vi "Register gRPC Messages.vi"(8 "error in (no error)":errorcluster, 11 "gRPC ID":T1) -> (0 "error out":errorcluster, 3 "gRPC ID Out":T1)   [LabVIEW 2021, in "CIF_PluginLoader_server.lvlib"]
uses:
  CIF_PluginLoader_server.lvlib
  <vilib>/gRPC/LabVIEW gRPC Library/Shared/grpcId.ctl
  <vilib>/gRPC/LabVIEW gRPC Library/Server API/typeDefs/Enum Metadata.ctl
  <vilib>/gRPC/LabVIEW gRPC Library/Server API/typeDefs/Message Metadata.ctl
  <vilib>/gRPC/LabVIEW gRPC Library/Server API/typeDefs/Message Element Metadata.ctl
  <vilib>/gRPC/LabVIEW gRPC Library/Server API/typeDefs/Message Element Type.ctl
  <vilib>/gRPC/LabVIEW gRPC Library/grpc-lvsupport-release.lvlib
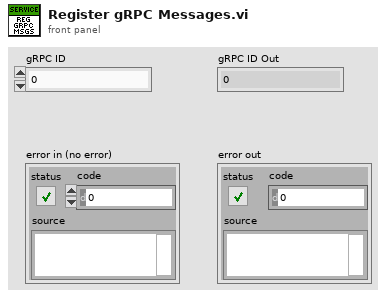
[diagram p1: front panel]
types:
  T1 = typedef "grpc-lvsupport-release.lvlib/grpcId.ctl" = u64
  T2 = typedef "grpc-lvsupport-release.lvlib/Enum Metadata.ctl" = cluster{"Version":i32, "Name":string, "Type Url":string, "Enum Values":string, "Allow Alias":bool}
  T3 = typedef "grpc-lvsupport-release.lvlib/Message Metadata.ctl" = cluster{"Version":i32, "Name":string, "Type Url":string, "Elements":T4[], "Has Oneof":bool}
  T4 = typedef "grpc-lvsupport-release.lvlib/Message Element Metadata.ctl" = cluster{"Field Name":string, "Embedded Message Name":string, "Protobuf Index":i32, "MessageElementType":T5, "Repeated":bool, "Is in Oneof":bool, "Oneof Container Name":string}
  T5 = typedef "grpc-lvsupport-release.lvlib/Message Element Type.ctl" = enum32{"Int32Value", "FloatValue", "DoubleValue", "BoolValue", "StringValue", "MessageValue", "Int64Value", "UInt32Value", "UInt64Value", "EnumValue", "Bytes", "Fixed64", "Fixed32", "SFixed64", "SFixed32", "SInt64", "SInt32"}
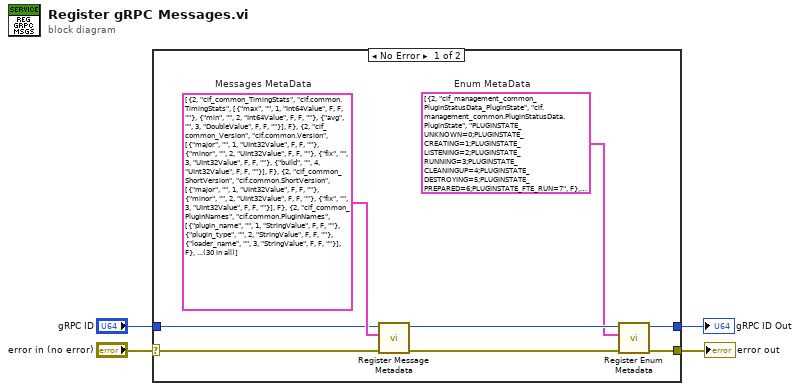
[diagram p0: block diagram]
diagram:
  n1 = case shown="No Error" "error in (no error)" {
    selector: "error in (no error)" -> [w10 w13]
    tunnel: [w9 w12] -> w2
    tunnel: [w6 w13] -> w1
    tunnel: "gRPC ID" -> [w9 w12]
    frame No Error {
      w5 = T2[] [{"Version"=2, "Name"="cif_management_common_PluginStatusData_PluginState", "Type Url"="cif.management_common.PluginStatusData.PluginState", "Enum Values"="PLUGINSTATE_UNKNOWN=0;PLUGINSTATE_CREATING=1;PLUGINSTATE_LISTENING=2;PLUGINSTATE_RUNNING=3;PLUGINSTATE_CLEANINGUP=4;PLUGINSTATE_DESTROYING=5;PLUGINSTATE_PREPARED=6;PLUGINSTATE_FTE_RUN=7", "Allow Alias"=FALSE}, {"Version"=2, "Name"="cif_management_common_ChannelDirection", "Type Url"="cif.management_common.ChannelDirection", "Enum Values"="CHANNELDIRECTION_UNKNOWN=0;CHANNELDIRECTION_PUBLISHER=1;CHANNELDIRECTION_SUBSCRIBER=2", "Allow Alias"=FALSE}, {"Version"=2, "Name"="cif_management_common_ChannelPattern", "Type Url"="cif.management_common.ChannelPattern", "Enum Values"="CHANNELPATTERN_UNKNOWN=0;CHANNELPATTERN_TAG=1;CHANNELPATTERN_FIFO=2;CHANNELPATTERN_MULTIFIFO=3;CHANNELPATTERN_BACKPRESSUREFIFO=4", "Allow Alias"=FALSE}, {"Version"=2, "Name"="cif_management_common_LoaderType", "Type Url"="cif.management_common.LoaderType", "Enum Values"="LOADERTYPE_UNKNOWN=0;LOADERTYPE_LABVIEW=1", "Allow Alias"=FALSE}]  # Enum MetaData
      w11 = T3[] [{"Version"=2, "Name"="cif_common_TimingStats", "Type Url"="cif.common.TimingStats", "Elements"=[{"Field Name"="max", "Embedded Message Name"="", "Protobuf Index"=1, "MessageElementType"=enum."Int64Value", "Repeated"=FALSE, "Is in Oneof"=FALSE, "Oneof Container Name"=""}, {"Field Name"="min", "Embedded Message Name"="", "Protobuf Index"=2, "MessageElementType"=enum."Int64Value", "Repeated"=FALSE, "Is in Oneof"=FALSE, "Oneof Container Name"=""}, {"Field Name"="avg", "Embedded Message Name"="", "Protobuf Index"=3, "MessageElementType"=enum."DoubleValue", "Repeated"=FALSE, "Is in Oneof"=FALSE, "Oneof Container Name"=""}], "Has Oneof"=FALSE}, {"Version"=2, "Name"="cif_common_Version", "Type Url"="cif.common.Version", "Elements"=[{"Field Name"="major", "Embedded Message Name"="", "Protobuf Index"=1, "MessageElementType"=enum."UInt32Value", "Repeated"=FALSE, "Is in Oneof"=FALSE, "Oneof Container Name"=""}, {"Field Name"="minor", "Embedded Message Name"="", "Protobuf Index"=2, "MessageElementType"=enum."UInt32Value", "Repeated"=FALSE, "Is in Oneof"=FALSE, "Oneof Container Name"=""}, {"Field Name"="fix", "Embedded Message Name"="", "Protobuf Index"=3, "MessageElementType"=enum."UInt32Value", "Repeated"=FALSE, "Is in Oneof"=FALSE, "Oneof Container Name"=""}, {"Field Name"="build", "Embedded Message Name"="", "Protobuf Index"=4, "MessageElementType"=enum."UInt32Value", "Repeated"=FALSE, "Is in Oneof"=FALSE, "Oneof Container Name"=""}], "Has Oneof"=FALSE}, {"Version"=2, "Name"="cif_common_ShortVersion", "Type Url"="cif.common.ShortVersion", "Elements"=[{"Field Name"="major", "Embedded Message Name"="", "Protobuf Index"=1, "MessageElementType"=enum."UInt32Value", "Repeated"=FALSE, "Is in Oneof"=FALSE, "Oneof Container Name"=""}, {"Field Name"="minor", "Embedded Message Name"="", "Protobuf Index"=2, "MessageElementType"=enum."UInt32Value", "Repeated"=FALSE, "Is in Oneof"=FALSE, "Oneof Container Name"=""}, {"Field Name"="fix", "Embedded Message Name"="", "Protobuf Index"=3, "MessageElementType"=enum."UInt32Value", "Repeated"=FALSE, "Is in Oneof"=FALSE, "Oneof Container Name"=""}], "Has Oneof"=FALSE}, {"Version"=2, "Name"="cif_common_PluginNames", "Type Url"="cif.common.PluginNames", "Elements"=[{"Field Name"="plugin_name", "Embedded Message Name"="", "Protobuf Index"=1, "MessageElementType"=enum."StringValue", "Repeated"=FALSE, "Is in Oneof"=FALSE, "Oneof Container Name"=""}, {"Field Name"="plugin_type", "Embedded Message Name"="", "Protobuf Index"=2, "MessageElementType"=enum."StringValue", "Repeated"=FALSE, "Is in Oneof"=FALSE, "Oneof Container Name"=""}, {"Field Name"="loader_name", "Embedded Message Name"="", "Protobuf Index"=3, "MessageElementType"=enum."StringValue", "Repeated"=FALSE, "Is in Oneof"=FALSE, "Oneof Container Name"=""}], "Has Oneof"=FALSE}, {"Version"=2, "Name"="cif_common_Status", "Type Url"="cif.common.Status", "Elements"=[{"Field Name"="code", "Embedded Message Name"="", "Protobuf Index"=1, "MessageElementType"=enum."Int32Value", "Repeated"=FALSE, "Is in Oneof"=FALSE, "Oneof Container Name"=""}, {"Field Name"="message", "Embedded Message Name"="", "Protobuf Index"=2, "MessageElementType"=enum."StringValue", "Repeated"=FALSE, "Is in Oneof"=FALSE, "Oneof Container Name"=""}], "Has Oneof"=FALSE}, {"Version"=2, "Name"="cif_common_Empty", "Type Url"="cif.common.Empty", "Elements"=[], "Has Oneof"=FALSE}, {"Version"=2, "Name"="cif_pluginloader_LoadPluginRequest", "Type Url"="cif.pluginloader.LoadPluginRequest", "Elements"=[{"Field Name"="plugin_name", "Embedded Message Name"="", "Protobuf Index"=1, "MessageElementType"=enum."StringValue", "Repeated"=FALSE, "Is in Oneof"=FALSE, "Oneof Container Name"=""}, {"Field Name"="path", "Embedded Message Name"="", "Protobuf Index"=2, "MessageElementType"=enum."StringValue", "Repeated"=FALSE, "Is in Oneof"=FALSE, "Oneof Container Name"=""}], "Has Oneof"=FALSE}, {"Version"=2, "Name"="cif_pluginloader_LoadPluginResponse", "Type Url"="cif.pluginloader.LoadPluginResponse", "Elements"=[{"Field Name"="status", "Embedded Message Name"="cif_common_Status", "Protobuf Index"=1, "MessageElementType"=enum."MessageValue", "Repeated"=FALSE, "Is in Oneof"=FALSE, "Oneof Container Name"=""}], "Has Oneof"=FALSE}, {"Version"=2, "Name"="cif_pluginloader_AbortPluginRequest", "Type Url"="cif.pluginloader.AbortPluginRequest", "Elements"=[{"Field Name"="plugin_name", "Embedded Message Name"="", "Protobuf Index"=1, "MessageElementType"=enum."StringValue", "Repeated"=FALSE, "Is in Oneof"=FALSE, "Oneof Container Name"=""}], "Has Oneof"=FALSE}, {"Version"=2, "Name"="cif_pluginloader_AbortPluginResponse", "Type Url"="cif.pluginloader.AbortPluginResponse", "Elements"=[{"Field Name"="status", "Embedded Message Name"="cif_common_Status", "Protobuf Index"=1, "MessageElementType"=enum."MessageValue", "Repeated"=FALSE, "Is in Oneof"=FALSE, "Oneof Container Name"=""}], "Has Oneof"=FALSE}, {"Version"=2, "Name"="cif_pluginloader_DestroyRequest", "Type Url"="cif.pluginloader.DestroyRequest", "Elements"=[], "Has Oneof"=FALSE}, {"Version"=2, "Name"="cif_pluginloader_DestroyResponse", "Type Url"="cif.pluginloader.DestroyResponse", "Elements"=[], "Has Oneof"=FALSE}, {"Version"=2, "Name"="cif_pluginloader_PingRequest", "Type Url"="cif.pluginloader.PingRequest", "Elements"=[], "Has Oneof"=FALSE}, {"Version"=2, "Name"="cif_pluginloader_PingResponse", "Type Url"="cif.pluginloader.PingResponse", "Elements"=[{"Field Name"="loader_info", "Embedded Message Name"="cif_management_common_LoaderInfoFull", "Protobuf Index"=1, "MessageElementType"=enum."MessageValue", "Repeated"=FALSE, "Is in Oneof"=FALSE, "Oneof Container Name"=""}], "Has Oneof"=FALSE}, {"Version"=2, "Name"="cif_pluginloader_DiscoverRequest", "Type Url"="cif.pluginloader.DiscoverRequest", "Elements"=[{"Field Name"="update_metadata", "Embedded Message Name"="", "Protobuf Index"=1, "MessageElementType"=enum."BoolValue", "Repeated"=FALSE, "Is in Oneof"=FALSE, "Oneof Container Name"=""}], "Has Oneof"=FALSE}, {"Version"=2, "Name"="cif_pluginloader_DiscoveredPlugin", "Type Url"="cif.pluginloader.DiscoveredPlugin", "Elements"=[{"Field Name"="file_path", "Embedded Message Name"="", "Protobuf Index"=1, "MessageElementType"=enum."StringValue", "Repeated"=FALSE, "Is in Oneof"=FALSE, "Oneof Container Name"=""}, {"Field Name"="file_name", "Embedded Message Name"="", "Protobuf Index"=2, "MessageElementType"=enum."StringValue", "Repeated"=FALSE, "Is in Oneof"=FALSE, "Oneof Container Name"=""}, {"Field Name"="plugin_type", "Embedded Message Name"="", "Protobuf Index"=3, "MessageElementType"=enum."StringValue", "Repeated"=FALSE, "Is in Oneof"=FALSE, "Oneof Container Name"=""}, {"Field Name"="plugin_version", "Embedded Message Name"="cif_common_Version", "Protobuf Index"=4, "MessageElementType"=enum."MessageValue", "Repeated"=FALSE, "Is in Oneof"=FALSE, "Oneof Container Name"=""}, {"Field Name"="plugin_metadata", "Embedded Message Name"="cif_management_common_PluginMetadata", "Protobuf Index"=5, "MessageElementType"=enum."MessageValue", "Repeated"=FALSE, "Is in Oneof"=FALSE, "Oneof Container Name"=""}, {"Field Name"="relative_path", "Embedded Message Name"="", "Protobuf Index"=6, "MessageElementType"=enum."StringValue", "Repeated"=TRUE, "Is in Oneof"=FALSE, "Oneof Container Name"=""}], "Has Oneof"=FALSE}, {"Version"=2, "Name"="cif_pluginloader_DiscoverResponse", "Type Url"="cif.pluginloader.DiscoverResponse", "Elements"=[{"Field Name"="discovered_plugins", "Embedded Message Name"="cif_pluginloader_DiscoveredPlugin", "Protobuf Index"=1, "MessageElementType"=enum."MessageValue", "Repeated"=TRUE, "Is in Oneof"=FALSE, "Oneof Container Name"=""}, {"Field Name"="status", "Embedded Message Name"="cif_common_Status", "Protobuf Index"=2, "MessageElementType"=enum."MessageValue", "Repeated"=FALSE, "Is in Oneof"=FALSE, "Oneof Container Name"=""}], "Has Oneof"=FALSE}, {"Version"=2, "Name"="cif_management_common_PluginMetadata", "Type Url"="cif.management_common.PluginMetadata", "Elements"=[{"Field Name"="description", "Embedded Message Name"="", "Protobuf Index"=1, "MessageElementType"=enum."StringValue", "Repeated"=FALSE, "Is in Oneof"=FALSE, "Oneof Container Name"=""}, {"Field Name"="history", "Embedded Message Name"="", "Protobuf Index"=2, "MessageElementType"=enum."StringValue", "Repeated"=FALSE, "Is in Oneof"=FALSE, "Oneof Container Name"=""}, {"Field Name"="author", "Embedded Message Name"="", "Protobuf Index"=3, "MessageElementType"=enum."StringValue", "Repeated"=FALSE, "Is in Oneof"=FALSE, "Oneof Container Name"=""}], "Has Oneof"=FALSE}, {"Version"=2, "Name"="cif_management_common_Channels", "Type Url"="cif.management_common.Channels", "Elements"=[{"Field Name"="channels", "Embedded Message Name"="cif_management_common_Channel", "Protobuf Index"=1, "MessageElementType"=enum."MessageValue", "Repeated"=TRUE, "Is in Oneof"=FALSE, "Oneof Container Name"=""}], "Has Oneof"=FALSE}, {"Version"=2, "Name"="cif_management_common_Channel", "Type Url"="cif.management_common.Channel", "Elements"=[{"Field Name"="name", "Embedded Message Name"="", "Protobuf Index"=1, "MessageElementType"=enum."StringValue", "Repeated"=FALSE, "Is in Oneof"=FALSE, "Oneof Container Name"=""}, {"Field Name"="direction", "Embedded Message Name"="cif_management_common_ChannelDirection", "Protobuf Index"=2, "MessageElementType"=enum."EnumValue", "Repeated"=FALSE, "Is in Oneof"=FALSE, "Oneof Container Name"=""}, {"Field Name"="type", "Embedded Message Name"="", "Protobuf Index"=3, "MessageElementType"=enum."StringValue", "Repeated"=FALSE, "Is in Oneof"=FALSE, "Oneof Container Name"=""}, {"Field Name"="custom_config", "Embedded Message Name"="", "Protobuf Index"=4, "MessageElementType"=enum."Bytes", "Repeated"=FALSE, "Is in Oneof"=FALSE, "Oneof Container Name"=""}, {"Field Name"="connected", "Embedded Message Name"="", "Protobuf Index"=5, "MessageElementType"=enum."BoolValue", "Repeated"=FALSE, "Is in Oneof"=FALSE, "Oneof Container Name"=""}, {"Field Name"="connected_name", "Embedded Message Name"="", "Protobuf Index"=6, "MessageElementType"=enum."StringValue", "Repeated"=FALSE, "Is in Oneof"=FALSE, "Oneof Container Name"=""}, {"Field Name"="forced", "Embedded Message Name"="", "Protobuf Index"=7, "MessageElementType"=enum."BoolValue", "Repeated"=FALSE, "Is in Oneof"=FALSE, "Oneof Container Name"=""}, {"Field Name"="channel_pattern", "Embedded Message Name"="cif_management_common_ChannelPattern", "Protobuf Index"=8, "MessageElementType"=enum."EnumValue", "Repeated"=FALSE, "Is in Oneof"=FALSE, "Oneof Container Name"=""}], "Has Oneof"=FALSE}, {"Version"=2, "Name"="cif_management_common_ChannelFilter", "Type Url"="cif.management_common.ChannelFilter", "Elements"=[{"Field Name"="name_regex", "Embedded Message Name"="", "Protobuf Index"=1, "MessageElementType"=enum."StringValue", "Repeated"=FALSE, "Is in Oneof"=FALSE, "Oneof Container Name"=""}, {"Field Name"="direction", "Embedded Message Name"="cif_management_common_ChannelDirection", "Protobuf Index"=2, "MessageElementType"=enum."EnumValue", "Repeated"=FALSE, "Is in Oneof"=FALSE, "Oneof Container Name"=""}, {"Field Name"="direction_filter", "Embedded Message Name"="", "Protobuf Index"=3, "MessageElementType"=enum."BoolValue", "Repeated"=FALSE, "Is in Oneof"=FALSE, "Oneof Container Name"=""}, {"Field Name"="type_regex", "Embedded Message Name"="", "Protobuf Index"=4, "MessageElementType"=enum."StringValue", "Repeated"=FALSE, "Is in Oneof"=FALSE, "Oneof Container Name"=""}, {"Field Name"="forced", "Embedded Message Name"="", "Protobuf Index"=5, "MessageElementType"=enum."BoolValue", "Repeated"=FALSE, "Is in Oneof"=FALSE, "Oneof Container Name"=""}, {"Field Name"="forced_filter", "Embedded Message Name"="", "Protobuf Index"=6, "MessageElementType"=enum."BoolValue", "Repeated"=FALSE, "Is in Oneof"=FALSE, "Oneof Container Name"=""}], "Has Oneof"=FALSE}, {"Version"=2, "Name"="cif_management_common_PluginStatusData", "Type Url"="cif.management_common.PluginStatusData", "Elements"=[{"Field Name"="state", "Embedded Message Name"="cif_management_common_PluginStatusData_PluginState", "Protobuf Index"=1, "MessageElementType"=enum."EnumValue", "Repeated"=FALSE, "Is in Oneof"=FALSE, "Oneof Container Name"=""}, {"Field Name"="timing_statistics", "Embedded Message Name"="cif_management_common_TimingStatistics", "Protobuf Index"=2, "MessageElementType"=enum."MessageValue", "Repeated"=FALSE, "Is in Oneof"=FALSE, "Oneof Container Name"=""}, {"Field Name"="fifo_statistics", "Embedded Message Name"="cif_management_common_FifoStatistics", "Protobuf Index"=3, "MessageElementType"=enum."MessageValue", "Repeated"=FALSE, "Is in Oneof"=FALSE, "Oneof Container Name"=""}, {"Field Name"="error", "Embedded Message Name"="cif_management_common_Error", "Protobuf Index"=4, "MessageElementType"=enum."MessageValue", "Repeated"=FALSE, "Is in Oneof"=FALSE, "Oneof Container Name"=""}, {"Field Name"="monitor_doubles", "Embedded Message Name"="cif_management_common_MonitorDoubles", "Protobuf Index"=5, "MessageElementType"=enum."MessageValue", "Repeated"=FALSE, "Is in Oneof"=FALSE, "Oneof Container Name"=""}, {"Field Name"="monitor_u64s", "Embedded Message Name"="cif_management_common_MonitorU64", "Protobuf Index"=6, "MessageElementType"=enum."MessageValue", "Repeated"=FALSE, "Is in Oneof"=FALSE, "Oneof Container Name"=""}, {"Field Name"="monitor_i64s", "Embedded Message Name"="cif_management_common_MonitorI64", "Protobuf Index"=7, "MessageElementType"=enum."MessageValue", "Repeated"=FALSE, "Is in Oneof"=FALSE, "Oneof Container Name"=""}], "Has Oneof"=FALSE}, {"Version"=2, "Name"="cif_management_common_TimingStatistics", "Type Url"="cif.management_common.TimingStatistics", "Elements"=[{"Field Name"="period", "Embedded Message Name"="cif_common_TimingStats", "Protobuf Index"=1, "MessageElementType"=enum."MessageValue", "Repeated"=FALSE, "Is in Oneof"=FALSE, "Oneof Container Name"=""}, {"Field Name"="wake_error", "Embedded Message Name"="cif_common_TimingStats", "Protobuf Index"=2, "MessageElementType"=enum."MessageValue", "Repeated"=FALSE, "Is in Oneof"=FALSE, "Oneof Container Name"=""}, {"Field Name"="execute", "Embedded Message Name"="cif_common_TimingStats", "Protobuf Index"=3, "MessageElementType"=enum."MessageValue", "Repeated"=FALSE, "Is in Oneof"=FALSE, "Oneof Container Name"=""}, {"Field Name"="housekeep", "Embedded Message Name"="cif_common_TimingStats", "Protobuf Index"=4, "MessageElementType"=enum."MessageValue", "Repeated"=FALSE, "Is in Oneof"=FALSE, "Oneof Container Name"=""}, {"Field Name"="idle", "Embedded Message Name"="cif_common_TimingStats", "Protobuf Index"=5, "MessageElementType"=enum."MessageValue", "Repeated"=FALSE, "Is in Oneof"=FALSE, "Oneof Container Name"=""}, {"Field Name"="cleanup", "Embedded Message Name"="cif_common_TimingStats", "Protobuf Index"=6, "MessageElementType"=enum."MessageValue", "Repeated"=FALSE, "Is in Oneof"=FALSE, "Oneof Container Name"=""}, {"Field Name"="custom_1", "Embedded Message Name"="cif_common_TimingStats", "Protobuf Index"=7, "MessageElementType"=enum."MessageValue", "Repeated"=FALSE, "Is in Oneof"=FALSE, "Oneof Container Name"=""}, {"Field Name"="custom_2", "Embedded Message Name"="cif_common_TimingStats", "Protobuf Index"=8, "MessageElementType"=enum."MessageValue", "Repeated"=FALSE, "Is in Oneof"=FALSE, "Oneof Container Name"=""}], "Has Oneof"=FALSE}, {"Version"=2, "Name"="cif_management_common_FifoStatistics", "Type Url"="cif.management_common.FifoStatistics", "Elements"=[{"Field Name"="from_t0", "Embedded Message Name"="cif_common_TimingStats", "Protobuf Index"=1, "MessageElementType"=enum."MessageValue", "Repeated"=FALSE, "Is in Oneof"=FALSE, "Oneof Container Name"=""}, {"Field Name"="from_previous_plugin", "Embedded Message Name"="cif_common_TimingStats", "Protobuf Index"=2, "MessageElementType"=enum."MessageValue", "Repeated"=FALSE, "Is in Oneof"=FALSE, "Oneof Container Name"=""}, {"Field Name"="output_error", "Embedded Message Name"="cif_common_TimingStats", "Protobuf Index"=3, "MessageElementType"=enum."MessageValue", "Repeated"=FALSE, "Is in Oneof"=FALSE, "Oneof Container Name"=""}], "Has Oneof"=FALSE}, {"Version"=2, "Name"="cif_management_common_MonitorDoubles", "Type Url"="cif.management_common.MonitorDoubles", "Elements"=[{"Field Name"="double_1", "Embedded Message Name"="", "Protobuf Index"=1, "MessageElementType"=enum."DoubleValue", "Repeated"=FALSE, "Is in Oneof"=FALSE, "Oneof Container Name"=""}, {"Field Name"="double_2", "Embedded Message Name"="", "Protobuf Index"=2, "MessageElementType"=enum."DoubleValue", "Repeated"=FALSE, "Is in Oneof"=FALSE, "Oneof Container Name"=""}, {"Field Name"="double_3", "Embedded Message Name"="", "Protobuf Index"=3, "MessageElementType"=enum."DoubleValue", "Repeated"=FALSE, "Is in Oneof"=FALSE, "Oneof Container Name"=""}, {"Field Name"="double_4", "Embedded Message Name"="", "Protobuf Index"=4, "MessageElementType"=enum."DoubleValue", "Repeated"=FALSE, "Is in Oneof"=FALSE, "Oneof Container Name"=""}], "Has Oneof"=FALSE}, {"Version"=2, "Name"="cif_management_common_MonitorU64", "Type Url"="cif.management_common.MonitorU64", "Elements"=[{"Field Name"="u64_1", "Embedded Message Name"="", "Protobuf Index"=1, "MessageElementType"=enum."UInt64Value", "Repeated"=FALSE, "Is in Oneof"=FALSE, "Oneof Container Name"=""}, {"Field Name"="u64_2", "Embedded Message Name"="", "Protobuf Index"=2, "MessageElementType"=enum."UInt64Value", "Repeated"=FALSE, "Is in Oneof"=FALSE, "Oneof Container Name"=""}, {"Field Name"="u64_3", "Embedded Message Name"="", "Protobuf Index"=3, "MessageElementType"=enum."UInt64Value", "Repeated"=FALSE, "Is in Oneof"=FALSE, "Oneof Container Name"=""}, {"Field Name"="u64_4", "Embedded Message Name"="", "Protobuf Index"=4, "MessageElementType"=enum."UInt64Value", "Repeated"=FALSE, "Is in Oneof"=FALSE, "Oneof Container Name"=""}], "Has Oneof"=FALSE}, {"Version"=2, "Name"="cif_management_common_MonitorI64", "Type Url"="cif.management_common.MonitorI64", "Elements"=[{"Field Name"="i64_1", "Embedded Message Name"="", "Protobuf Index"=1, "MessageElementType"=enum."Int64Value", "Repeated"=FALSE, "Is in Oneof"=FALSE, "Oneof Container Name"=""}, {"Field Name"="i64_2", "Embedded Message Name"="", "Protobuf Index"=2, "MessageElementType"=enum."Int64Value", "Repeated"=FALSE, "Is in Oneof"=FALSE, "Oneof Container Name"=""}, {"Field Name"="i64_3", "Embedded Message Name"="", "Protobuf Index"=3, "MessageElementType"=enum."Int64Value", "Repeated"=FALSE, "Is in Oneof"=FALSE, "Oneof Container Name"=""}, {"Field Name"="i64_4", "Embedded Message Name"="", "Protobuf Index"=4, "MessageElementType"=enum."Int64Value", "Repeated"=FALSE, "Is in Oneof"=FALSE, "Oneof Container Name"=""}], "Has Oneof"=FALSE}, {"Version"=2, "Name"="cif_management_common_Error", "Type Url"="cif.management_common.Error", "Elements"=[{"Field Name"="status", "Embedded Message Name"="", "Protobuf Index"=1, "MessageElementType"=enum."BoolValue", "Repeated"=FALSE, "Is in Oneof"=FALSE, "Oneof Container Name"=""}, {"Field Name"="code", "Embedded Message Name"="", "Protobuf Index"=2, "MessageElementType"=enum."Int32Value", "Repeated"=FALSE, "Is in Oneof"=FALSE, "Oneof Container Name"=""}], "Has Oneof"=FALSE}, {"Version"=2, "Name"="cif_management_common_LoaderInfo", "Type Url"="cif.management_common.LoaderInfo", "Elements"=[{"Field Name"="loader_type", "Embedded Message Name"="cif_management_common_LoaderType", "Protobuf Index"=1, "MessageElementType"=enum."EnumValue", "Repeated"=FALSE, "Is in Oneof"=FALSE, "Oneof Container Name"=""}, {"Field Name"="loader_name", "Embedded Message Name"="", "Protobuf Index"=2, "MessageElementType"=enum."StringValue", "Repeated"=FALSE, "Is in Oneof"=FALSE, "Oneof Container Name"=""}], "Has Oneof"=FALSE}, {"Version"=2, "Name"="cif_management_common_LoaderInfoFull", "Type Url"="cif.management_common.LoaderInfoFull", "Elements"=[{"Field Name"="loader_type", "Embedded Message Name"="cif_management_common_LoaderType", "Protobuf Index"=1, "MessageElementType"=enum."EnumValue", "Repeated"=FALSE, "Is in Oneof"=FALSE, "Oneof Container Name"=""}, {"Field Name"="loader_name", "Embedded Message Name"="", "Protobuf Index"=2, "MessageElementType"=enum."StringValue", "Repeated"=FALSE, "Is in Oneof"=FALSE, "Oneof Container Name"=""}, {"Field Name"="grpc_port", "Embedded Message Name"="", "Protobuf Index"=3, "MessageElementType"=enum."Int32Value", "Repeated"=FALSE, "Is in Oneof"=FALSE, "Oneof Container Name"=""}, {"Field Name"="pid", "Embedded Message Name"="", "Protobuf Index"=4, "MessageElementType"=enum."UInt32Value", "Repeated"=FALSE, "Is in Oneof"=FALSE, "Oneof Container Name"=""}], "Has Oneof"=FALSE}]  # Messages MetaData
      n2 = call <vilib>:"Register Message Metadata.vi"("error in"=w10, "Messages"=w11, "gRPCid in"=w9) -> ("error out"=w7:errorcluster, "gRPCid out"=w8:T1)  [unwired: 7 in]
      n3 = call <vilib>:"Register Enum Metadata.vi"("error in"=w7, "Enum Metadata"=w5, "gRPCid in"=w8) -> ("error out"=w6:errorcluster)  [unwired: 7 in, 1 out]
    }
    frame Error {
    }
  }
  "error out" <- w1
  "gRPC ID Out" <- w2
